vi "Phase and Amplitude Matching.vi"() -> ()   [LabVIEW 2012]
uses:
  <vilib>/measure/NI_MAPro.lvlib
  <vilib>/measure/matone.llb/Extract Single Tone Information 1 Chan.vi
  <vilib>/measure/NI_MABase.lvlib
  <vilib>/measure/maresamp.llb/Align two Waveforms (continuous).vi
panel:
  out "Processed Waveforms":waveform(dbl)[](graph)=[{"t0"=timestamp(0 s since 1904-01-01), "dt"=0.001, "Y"=array[961 elements]}, {"t0"=timestamp(0 s since 1904-01-01), "dt"=0.001, "Y"=array[961 elements]}]
  in  "Enable Phase Match?":bool=TRUE
  in  "Enable Amplitude Match?":bool=TRUE
  in  "Sampling Info A":cluster{"Fs":dbl, "#s":dbl}={"Fs"=1000.0, "#s"=1000.0}
  in  "Phase A":dbl=45.0
  in  "Amplitude A":dbl=5.0
  in  "Sampling Info B":cluster{"Fs":dbl, "#s":dbl}={"Fs"=1000.0, "#s"=1000.0}
  in  "Phase B":dbl=180.0
  in  "Amplitude B":dbl=1.0
  in  "Waveform Frequency":dbl=10.0
  out "Original Waveforms":waveform(dbl)[](graph)=[{"t0"=timestamp(0 s since 1904-01-01), "dt"=0.001, "Y"=array[1000 elements]}, {"t0"=timestamp(0 s since 1904-01-01), "dt"=0.001, "Y"=array[1000 elements]}]
  # "Waveform A Properties"
  # "Waveform B Properties"
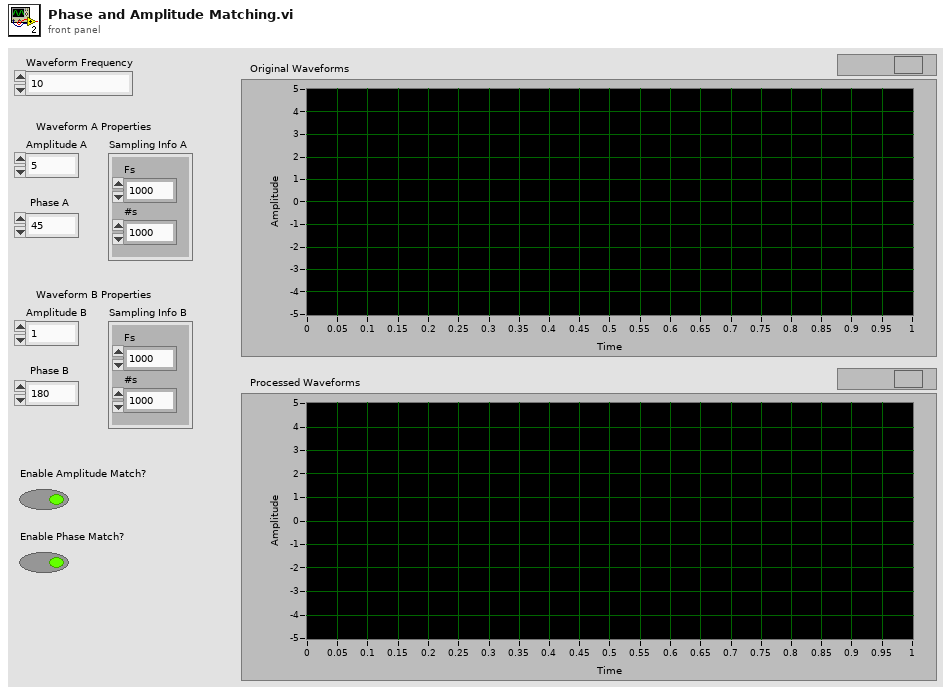
[diagram p1: front panel]
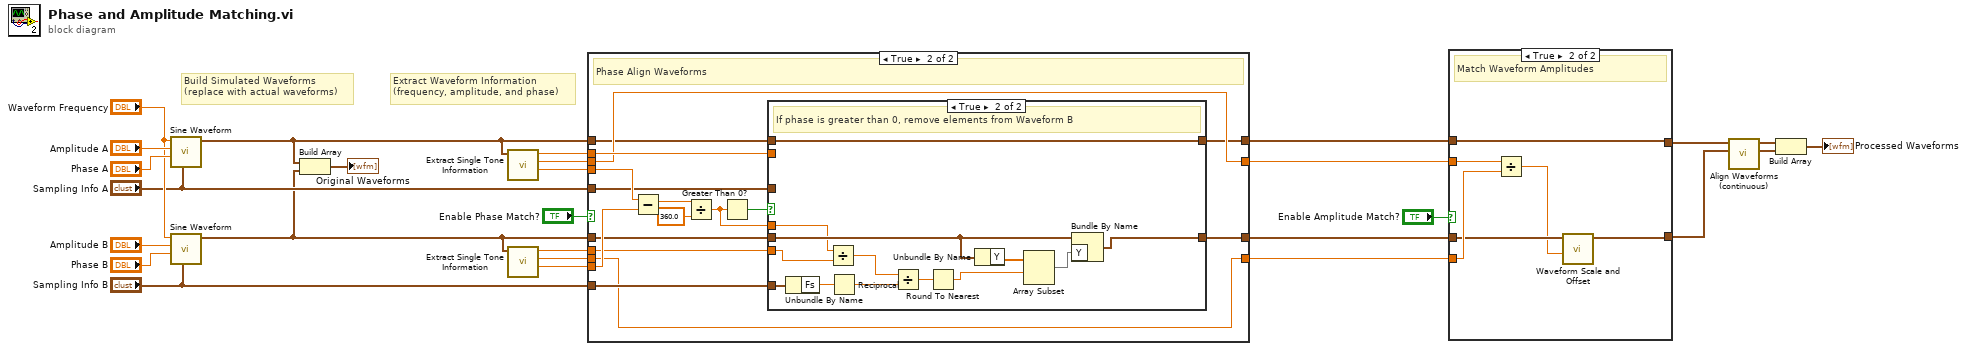
[diagram p0: block diagram]
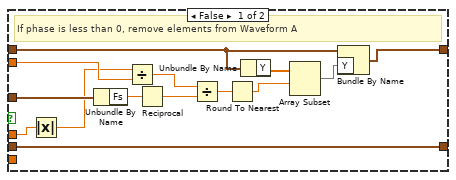
[diagram p4: hidden frame]
diagram:
  # "Extract Waveform Information\n(frequency, amplitude, and phase)"
  # "Build Simulated Waveforms\n(replace with actual waveforms)"
  n1 = call <vilib>:"Sine Waveform.vi"("sampling info"="Sampling Info A", "phase"="Phase A", "amplitude"="Amplitude A", "frequency"="Waveform Frequency") -> ("signal out"=w12:waveform(dbl))  [unwired: 6 in, 1 out]
  n2 = call <vilib>:"Sine Waveform.vi"("sampling info"="Sampling Info B", "phase"="Phase B", "amplitude"="Amplitude B", "frequency"="Waveform Frequency") -> ("signal out"=w16:waveform(dbl))  [unwired: 6 in, 1 out]
  n3 = Build Array(w12, w16) -> (→"Original Waveforms":waveform(dbl)[])
  n4 = call-poly <vilib>:"Extract Single Tone Information.vi"("time signal in"=w12) -> ("detected phase (deg)"=w17:dbl, "detected amplitude"=w18:dbl, "detected frequency"=w19:dbl)  [unwired: 5 in, 3 out]
  n5 = call-poly <vilib>:"Extract Single Tone Information.vi"("time signal in"=w16) -> ("detected phase (deg)"=w13:dbl, "detected amplitude"=w14:dbl, "detected frequency"=w15:dbl)  [unwired: 5 in, 3 out]
  n6 = case shown="True" "Enable Phase Match?" {
    tunnel: "Sampling Info A" -> [_ w41]
    tunnel: "Sampling Info B" -> [_ w42]
    tunnel: w12 -> [w28 w36]
    tunnel: w19 -> [_ w40]
    tunnel: w18 -> [w31 w38]
    tunnel: w17 -> [_ w47]
    tunnel: w16 -> [w29 w35]
    tunnel: w15 -> [_ w39]
    tunnel: w14 -> [w30 w37]
    tunnel: w13 -> [_ w46]
    tunnel: [w31 w38] -> w7
    tunnel: [w30 w37] -> w6
    tunnel: [w28 w33] -> w8
    tunnel: [w29 w32] -> w9
    frame False {
      # "Skip Phase Alignment"
    }
    frame True {
      # "Phase Align Waveforms"
      n7 = Subtract(x=w47, y=w46) -> (x-y=w45:dbl)
      n8 = Divide(x=w45, y=360.0) -> (x/y=w34:dbl)
      n9 = Greater Than 0?(x=w34) -> (x > 0?=w43:bool)
      n10 = case shown="True" w43 {
        tunnel: w42 -> [_ w74]
        tunnel: w41 -> [w56 _]
        tunnel: w40 -> [w50 _]
        tunnel: w39 -> [_ w63]
        tunnel: w36 -> [w53 w65]
        tunnel: w35 -> [w61 w69]
        tunnel: w34 -> [w49 w62]
        tunnel: [w51 w65] -> w33
        tunnel: [w61 w64] -> w32
        frame False {
          # "If phase is less than 0, remove elements from Waveform A"
          n11 = Absolute Value(x=w49) -> (abs(x)=w48:dbl)
          n12 = Unbundle By Name(w56) -> ("Fs"=w57:dbl)
          n13 = Divide(x=w48, y=w50) -> (x/y=w58:dbl)
          n14 = Reciprocal(x=w57) -> (1/x=w59:dbl)
          n15 = Divide(x=w58, y=w59) -> (x/y=w60:dbl)
          n16 = Round To Nearest(number=w60) -> (nearest integer value=w52:dbl)
          n17 = Unbundle By Name(w53) -> ("Y"=w54:dbl[])
          n18 = Array Subset(array=w54, index=w52) -> (w55:dbl[])  [unwired: 1 in]
          n19 = Bundle By Name(cluster=w53, "Y"=w55) -> (w51:waveform(dbl))
        }
        frame True {
          # "If phase is greater than 0, remove elements from Waveform B"
          n20 = Unbundle By Name(w74) -> ("Fs"=w73:dbl)
          n21 = Divide(x=w62, y=w63) -> (x/y=w72:dbl)
          n22 = Reciprocal(x=w73) -> (1/x=w71:dbl)
          n23 = Divide(x=w72, y=w71) -> (x/y=w67:dbl)
          n24 = Round To Nearest(number=w67) -> (nearest integer value=w66:dbl)
          n25 = Unbundle By Name(w69) -> ("Y"=w70:dbl[])
          n26 = Array Subset(array=w70, index=w66) -> (w68:dbl[])  [unwired: 1 in]
          n27 = Bundle By Name(cluster=w69, "Y"=w68) -> (w64:waveform(dbl))
        }
      }
    }
  }
  n28 = case shown="True" "Enable Amplitude Match?" {
    tunnel: w9 -> [w75 w80]
    tunnel: w8 -> [w76 w77]
    tunnel: w7 -> [_ w82]
    tunnel: w6 -> [_ w81]
    tunnel: [w76 w77] -> w5
    tunnel: [w75 w79] -> w4
    frame False {
      # "Skip Amplitude Matching"
    }
    frame True {
      # "Match Waveform Amplitudes"
      n29 = Divide(x=w82, y=w81) -> (x/y=w78:dbl)
      n30 = call <vilib>:"Waveform Scale and Offset.vi"("scale"=w78, "waveform in"=w80) -> ("waveform out"=w79:waveform(dbl))  [unwired: 8 in, 1 out]
    }
  }
  n31 = call-poly <vilib>:"Align Waveforms (continuous).vi"("waveform B in"=w4, "waveform A in"=w5) -> ("waveform B out"=w2:waveform(dbl), "waveform A out"=w3:waveform(dbl))  [unwired: 7 in, 1 out]
  n32 = Build Array(w3, w2) -> (→"Processed Waveforms":waveform(dbl)[])
